vi "Do Charact.vi"(0 "Vector Path in":refnum<class "Vector Path.lvclass">, 5 "Standard Type":T1, 11 "error in (no error)":errorcluster) -> (4 "Vector Path out":refnum<class "Vector Path.lvclass">, 6 "Aborted":bool, 15 "error out":errorcluster)   [LabVIEW 2023, in "RFFixtureCharact.Public.lvlib" / "Vector Path.lvclass"]
uses:
  Vector Path.lvclass
  Vector Path.lvclass/Vector Path.ctl
  Instruments/Cal Standard/Type Definitions/Standard Type.ctl
  Instruments/RFFixtureCharact.Instruments.lvlib
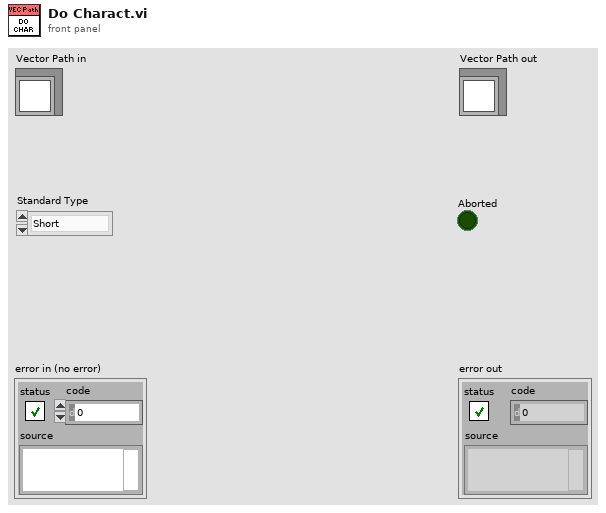
[diagram p1: front panel]
types:
  T1 = typedef "RFFixtureCharact.Instruments.lvlib/Standard Type.ctl" = enum16{"Short", "Open", "Load", "PowerMeter", "None"}
  T2 = typedef "RFFixtureCharact.Instruments.lvlib/One-Port Charact Data.ctl" = cluster{"Standard Type":T1, "Frequencies":dbl[], "S11":cdb[]}
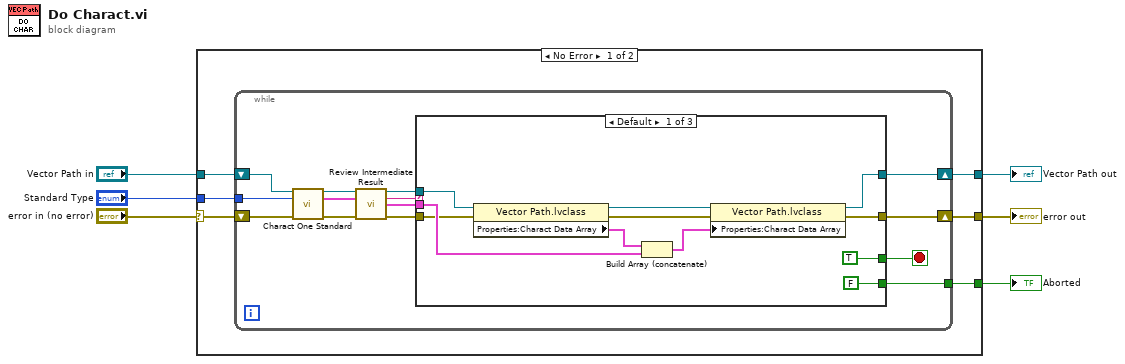
[diagram p0: block diagram]
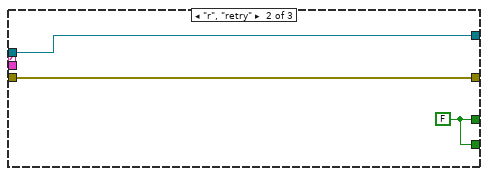
[diagram p2: hidden frame]
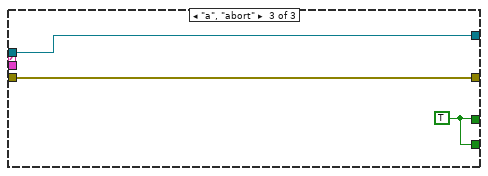
[diagram p3: hidden frame]
diagram:
  n1 = case shown="No Error" "error in (no error)" {
    selector: "error in (no error)" -> [w7 w45]
    tunnel: "Vector Path in" -> [w8 w44]
    tunnel: [w11 w45] -> w4
    tunnel: [w12 w44] -> w3
    tunnel: "Standard Type" -> [w9 _]
    tunnel: [w10 _] -> w1
    frame No Error {
      n2 = while {
        shift-right: [w19] -> w11
        shift-left: w7 -> [w26]
        shift-right: [w21] -> w12
        shift-left: w8 -> [w25]
        tunnel: [w22] -> w10
        tunnel: w9 -> [w18]
        stop <- w23 stop-if-true
        n3 = call-dynamic "Charact One Standard.vi"("Vector Path in"=w25, "Standard Type"=w18, "error in"=w26) -> ("Vector Path out"=w15:refnum<class "Vector Path.lvclass">, "One-Port Charact Data"=w13:T2, "error out"=w24:errorcluster)  [unwired: 10 in]
        n4 = call-dynamic "Review Intermediate Result.vi"("Vector 26GHz Path in"=w15, "One-Port Charact Data In"=w13, "error in (no error)"=w24) -> ("Vector 26GHz Path out"=w14:refnum<class "Vector Path.lvclass">, "Response"=w17:string, "One-Port Charact Data Out"=w16:T2, "error out"=w20:errorcluster)  [unwired: 9 in]
        n5 = case shown="Default" w17 {
          tunnel: [TRUE w38 w41] -> w23
          tunnel: [FALSE w38 w41] -> w22
          tunnel: [w28 w40 w43] -> w21
          tunnel: w14 -> [w35 w40 w43]
          tunnel: w20 -> [w34 w39 w42]
          tunnel: [w33 w39 w42] -> w19
          tunnel: w16 -> [w36 _ _]
          frame Default {
            n6 = property class="Vector Path.lvclass"(reference=w35, error in=w34) -> (reference out=w31:refnum<class "Vector Path.lvclass">, error out=w29:errorcluster, "Properties:Charact Data Array"=w32:T2[])
            n7 = Build Array (concatenate)(w32, w36) -> (w30:T2[])
            n8 = property class="Vector Path.lvclass"(reference=w31, error in=w29, "Properties:Charact Data Array"=w30) -> (reference out=w28:refnum<class "Vector Path.lvclass">, error out=w33:errorcluster)
          }
          frame "r", "retry" {
            w38 = FALSE
          }
          frame "a", "abort" {
            w41 = TRUE
          }
        }
      }
    }
    frame Error {
    }
  }
  "error out" <- w4
  "Vector Path out" <- w3
  "Aborted" <- w1
